vi "DMM_Mixed Meas Close.vi"(0 "DMM Handle In":refnum<k15>, 11 "error in":errorcluster) -> (15 "error out":errorcluster)   [LabVIEW 2021, in "DMM_Mixed Measurement.lvlib"]
doc: "Closes the NI-DMM session specifed in DMM Handle In and releases the resource."
uses:
  DMM_Mixed Measurement.lvlib
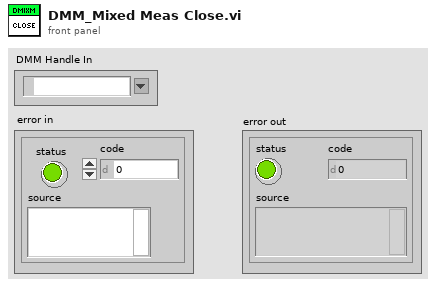
[diagram p1: front panel]
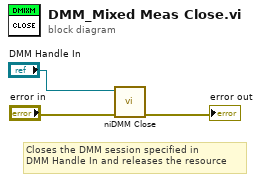
[diagram p0: block diagram]
diagram:
  # "Closes the DMM session specified in \nDMM Handle In and releases the resource"
  n1 = call <instrlib>:"niDMM Close.vi"("error in (no error)"="error in", "instrument handle"="DMM Handle In") -> ("error out"=→"error out":errorcluster)  [unwired: 9 in]
